vi "low energy end.vi"() -> ()   [LabVIEW 2016, in "beamline sections.lvlib"]
uses:
  beamline sections.lvlib
panel:
  out "error out":errorcluster
  out "Steerer Y":dbl format="%#_4g"
  in  "Tab Control":enum32{"Controls", "readbacks"}(tab)
  in  "Low Energy Einzel":dbl(slide) scale=30.0..50.0
  in  "Injector Image Einzel":dbl(slide) scale=30.0..50.0
  out "Low Energy Einzel Display":bool=TRUE
  out "Tank Entrance  Steerer Display":bool
  out "Low energy waist Steerer Display":bool=TRUE
  out "Injector Image Steerer display":bool
  out "Injector image Einzel Display":bool=TRUE
  in  "Tank Entrance Y2 steerer":dbl(slide) scale=-3.0..3.0
  in  "Tank Entrance Y1 steerer":dbl(slide) scale=-3.0..3.0
  in  "Tank Entrance  X steerer":dbl(slide) scale=-3.0..3.0
  in  "Low Energy Waist Y steerer":dbl(slide) scale=-1.0..1.0
  in  "Low Energy Waist  X steerer":dbl(slide) scale=-1.0..1.0
  in  "Injector Image Y steerer":dbl(slide) scale=-1.0..1.0
  in  "Injector Image X steerer":dbl(slide) scale=-1.0..1.0
  out "Low Energy Einzel Voltage":dbl format="%#.2g"
  out "Low Energy Einzel Current":dbl format="%#.2g"
  out "Tank Exit  X V":dbl format="%#.2g"
  out "Tank Exit Y #1 V":dbl format="%#.2g"
  out "Tank Exit Y #2 V":dbl format="%#.2g"
  out "Low energy waist  X V":dbl format="%#.2g"
  out "Low energy waist  Y V":dbl format="%#.2g"
  out "Inj image Einzel Current":dbl format="%#.2g"
  out "Inj image Einzel":dbl format="%#.2g"
  out "Inj Image X Voltage":dbl format="%#.2g"
  out "Inj Image Y Voltage":dbl format="%#.2g"
  in  "stop":bool
  out "LE Waist  Ion gauge Cluster":T1
  out "Tank entrance Ion gauge Cluster 1":T1
  out "Low energy   Y-":dbl format="%#_4g"
  out "Low energy   Y+":dbl format="%#_4g"
  out "Low energy   X-":dbl format="%#_4g"
  out "Low energy   X+":dbl format="%#_4g"
  out "Low energy   Y-  2":dbl format="%#_4g"
  out "Low energy   Y+  2":dbl format="%#_4g"
  out "Low energy   X-  V":dbl format="%#_4g"
  out "Low energy   X+  V":dbl format="%#_4g"
  out "Low energy waist  X+":dbl format="%#_4g"
  out "Low energy waist  Y- V":dbl format="%#_4g"
  out "Low energy waist  Y+ V":dbl format="%#_4g"
  out "Low energy waist  X- V":dbl format="%#_4g"
  out "Low energy waist  X+ V":dbl format="%#_4g"
  in  "Injector image Y  -":dbl format="%#_4g"
  in  "Injector image Y +":dbl format="%#_4g"
  in  "Injector image X  -":dbl format="%#_4g"
  in  "Injector image X +":dbl format="%#_4g"
  out "Injector image Y  -  V":dbl format="%#_4g"
  out "Injector image Y +   V":dbl format="%#_4g"
  out "Injector image X  - V":dbl format="%#_4g"
  out "Injector image X +  V":dbl format="%#_4g"
  out "Low energy   Y+ 2  V":dbl format="%#_4g"
  out "Low energy   Y- 2  V":dbl format="%#_4g"
  out "Tank entrance Cryo pump":T2
  out "Low energy   Y+  V":dbl format="%#_4g"
  out "Low energy   Y-  V":dbl format="%#_4g"
  out "Low energy waist  X-":dbl format="%#_4g"
  out "Low energy waist  Y+":dbl format="%#_4g"
  out "Low energy waist  Y-":dbl format="%#_4g"
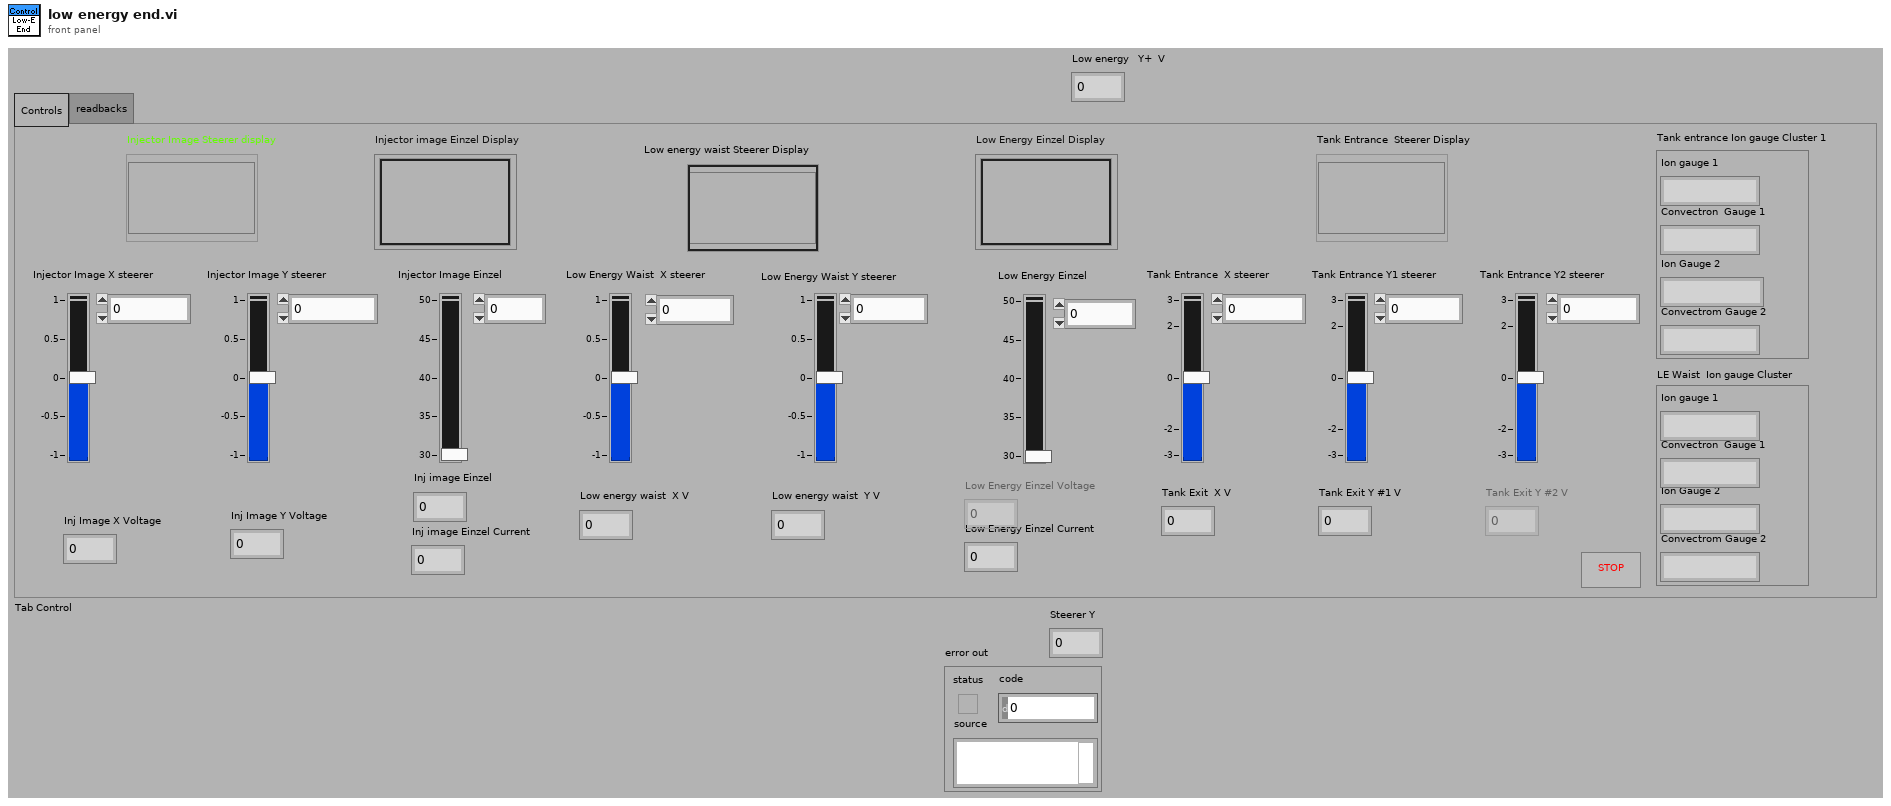
[diagram p1: front panel]
types:
  T1 = cluster{"Ion gauge 1":string, "Convectron  Gauge 1 ":string, "Ion Gauge 2":string, "Convectrom Gauge 2":string}
  T2 = cluster{"First Stage":dbl, "Second stage":dbl, "Hours since last regen":dbl, "Pump ON":bool, "Time on":dbl}
  T3 = typedef "saveload.ctl" = cluster{"OK Button":bool, "OK Button 2":bool, "OK Button 3":bool, "OK Button 4":bool}
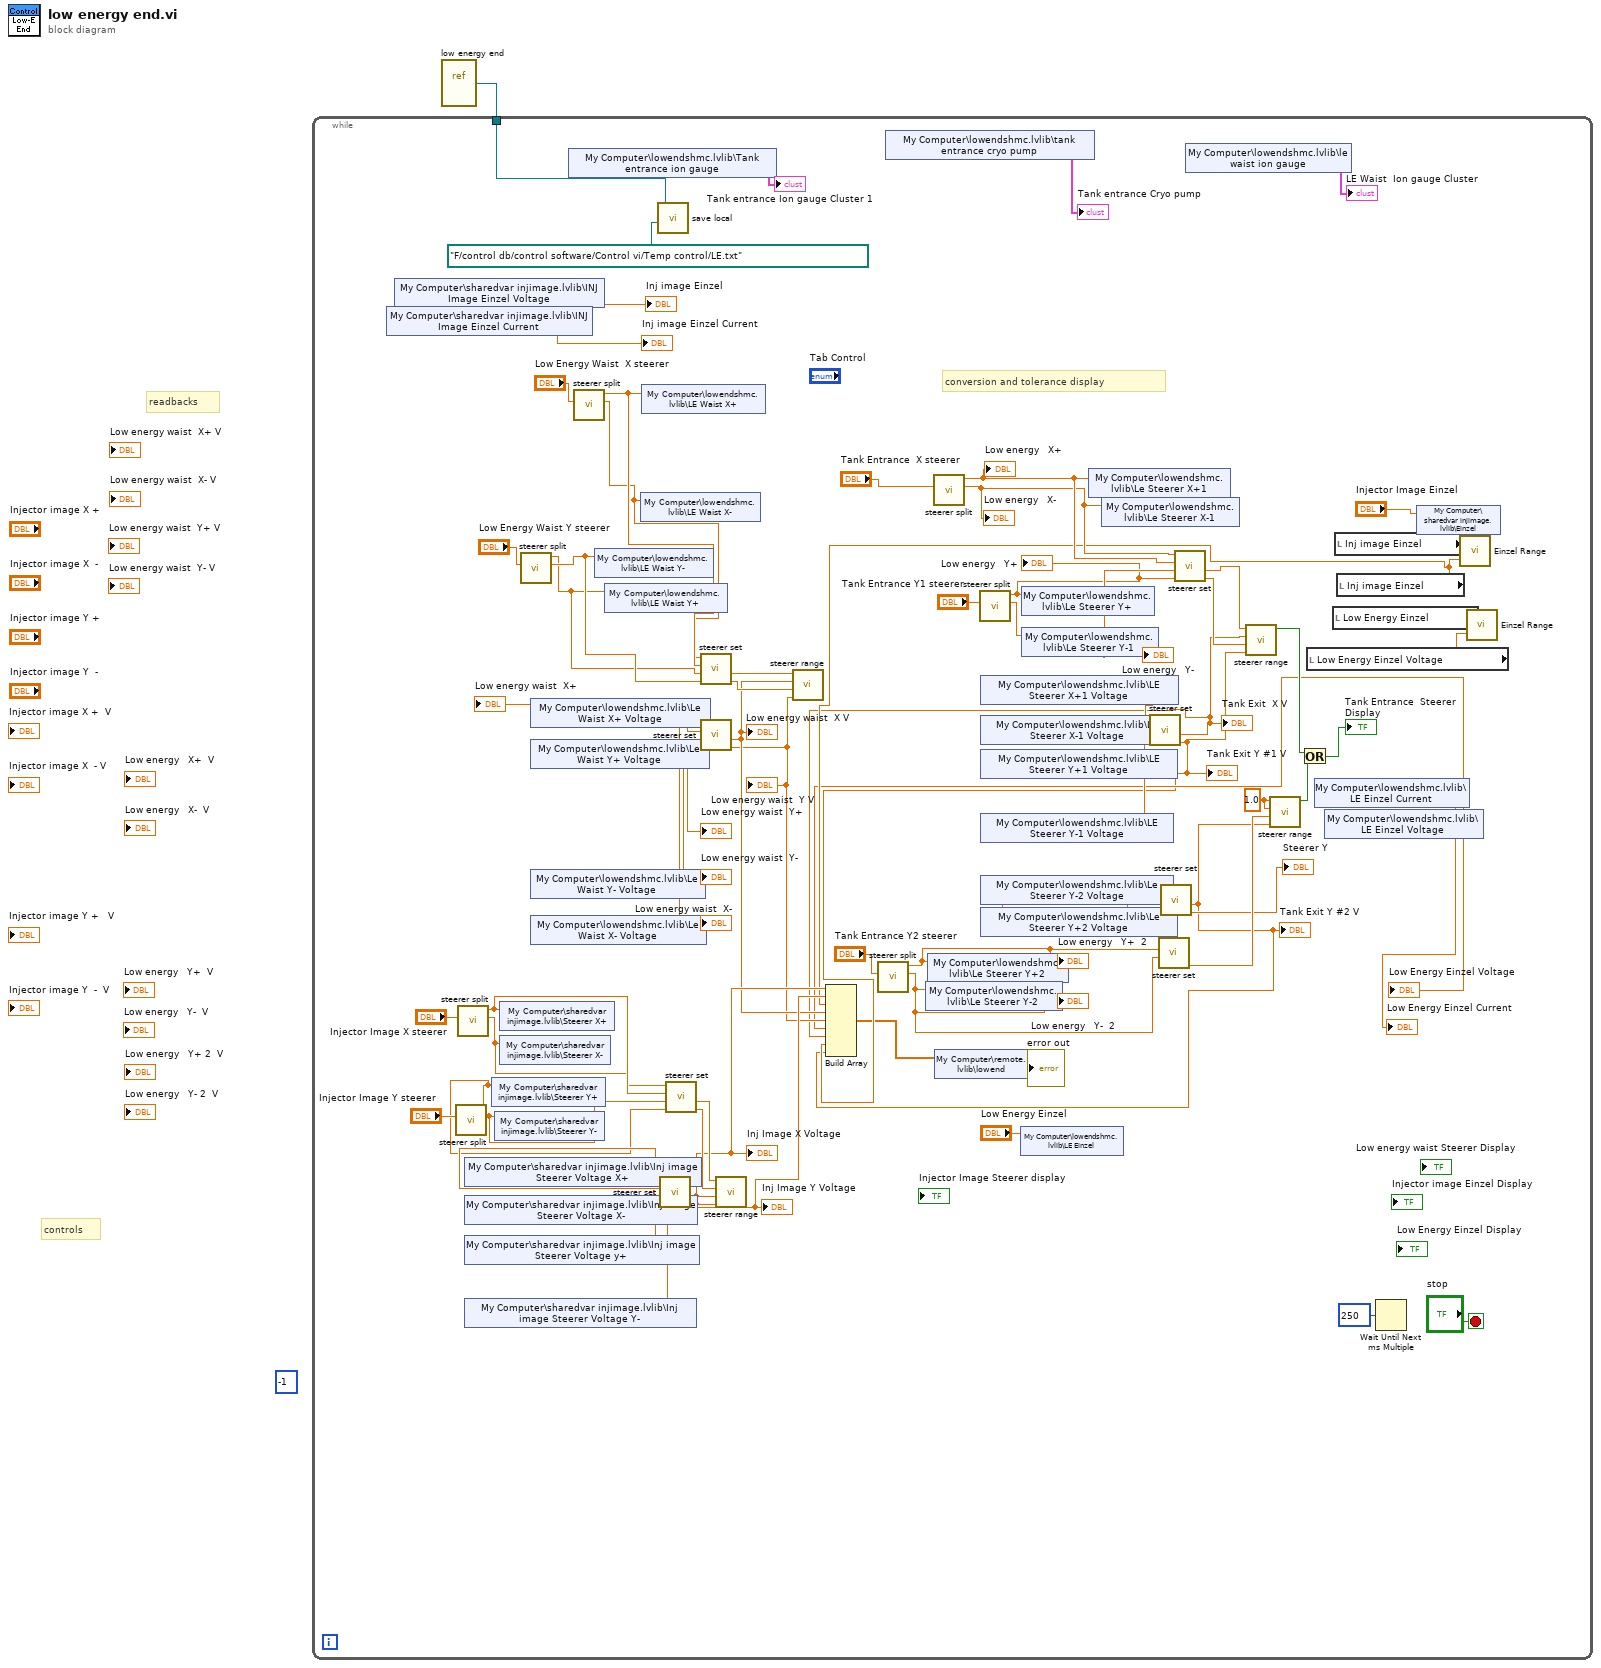
[diagram p0: block diagram]
diagram:
  (unwired) -1 ("index of element")
  # "readbacks"
  # "controls"
  n1 = vi-ref "low energy end.vi"() -> (w1:refnum<vi>)
  n2 = while {
    tunnel: w1 -> [w58]
    stop <- "stop" stop-if-true
    w66 = 1.0 ("Steerer X Set")
    # "conversion and tolerance display"
    n3 = shared-variable "My Computer\\sharedvar injimage.lvlib\\INJ Image Einzel Current"() -> (→"Inj image Einzel Current":dbl)  [unwired: 1 in, 1 out]
    n4 = shared-variable "My Computer\\sharedvar injimage.lvlib\\INJ Image Einzel Voltage"() -> (→"Inj image Einzel":dbl)  [unwired: 1 in, 1 out]
    n5 = call "steerer split.vi"("Steerer in"="Injector Image Y steerer") -> ("Steerer +"=w24:dbl, "Steerer -"=w23:dbl)  [unwired: 7 out]
    n6 = call "steerer split.vi"("Steerer in"="Injector Image X steerer") -> ("Steerer +"=w26:dbl, "Steerer -"=w25:dbl)  [unwired: 7 out]
    n7 = shared-variable "My Computer\\sharedvar injimage.lvlib\\Inj image Steerer Voltage X+"() -> (w35:dbl)  [unwired: 1 in, 1 out]
    n8 = shared-variable "My Computer\\sharedvar injimage.lvlib\\Inj image Steerer Voltage X-"() -> (w34:dbl)  [unwired: 1 in, 1 out]
    n9 = shared-variable "My Computer\\sharedvar injimage.lvlib\\Inj image Steerer Voltage y+"() -> (w33:dbl)  [unwired: 1 in, 1 out]
    n10 = shared-variable "My Computer\\sharedvar injimage.lvlib\\Inj image Steerer Voltage Y-"() -> (w36:dbl)  [unwired: 1 in, 1 out]
    n11 = shared-variable "My Computer\\sharedvar injimage.lvlib\\Steerer Y+"(w24) -> ()  [unwired: 1 in, 1 out]
    n12 = shared-variable "My Computer\\sharedvar injimage.lvlib\\Steerer Y-"(w23) -> ()  [unwired: 1 in, 1 out]
    n13 = shared-variable "My Computer\\sharedvar injimage.lvlib\\Steerer X+"(w26) -> ()  [unwired: 1 in, 1 out]
    n14 = shared-variable "My Computer\\sharedvar injimage.lvlib\\Steerer X-"(w25) -> ()  [unwired: 1 in, 1 out]
    n15 = call "steerer split.vi"("Steerer in"="Low Energy Waist Y steerer") -> ("Steerer +"=w31:dbl, "Steerer -"=w32:dbl)  [unwired: 7 out]
    n16 = shared-variable "My Computer\\lowendshmc.lvlib\\Le Waist X+ Voltage"() -> (w40:dbl)  [unwired: 1 in, 1 out]
    "Low energy waist  X+" <- w40
    n17 = shared-variable "My Computer\\lowendshmc.lvlib\\Le Waist Y+ Voltage"() -> (w38:dbl)  [unwired: 1 in, 1 out]
    "Low energy waist  Y+" <- w38
    n18 = shared-variable "My Computer\\lowendshmc.lvlib\\Le Waist Y- Voltage"() -> (w37:dbl)  [unwired: 1 in, 1 out]
    "Low energy waist  Y-" <- w37
    n19 = shared-variable "My Computer\\lowendshmc.lvlib\\Le Waist X- Voltage"() -> (w39:dbl)  [unwired: 1 in, 1 out]
    "Low energy waist  X-" <- w39
    n20 = shared-variable "My Computer\\lowendshmc.lvlib\\Tank entrance ion gauge"() -> (→"Tank entrance Ion gauge Cluster 1":cluster{string, string, string, string})  [unwired: 1 in, 1 out]
    n21 = call "steerer split.vi"("Steerer in"="Low Energy Waist  X steerer") -> ("Steerer +"=w30:dbl, "Steerer -"=w29:dbl)  [unwired: 7 out]
    n22 = shared-variable "My Computer\\lowendshmc.lvlib\\LE Waist Y-"(w32) -> ()  [unwired: 1 in, 1 out]
    n23 = shared-variable "My Computer\\lowendshmc.lvlib\\LE Waist Y+"(w31) -> ()  [unwired: 1 in, 1 out]
    n24 = shared-variable "My Computer\\lowendshmc.lvlib\\LE Waist X-"(w29) -> ()  [unwired: 1 in, 1 out]
    n25 = shared-variable "My Computer\\lowendshmc.lvlib\\LE Waist X+"(w30) -> ()  [unwired: 1 in, 1 out]
    n26 = call "save local.vi"("file path (use dialog)"=path "F:/control db/control software/Control vi/Temp control/LE.txt", "VI Refnum"=w58) -> ("Ring"=w61:T3)  [unwired: 2 out]
    n27 = call "steerer set.vi"("Injector image X  -"=w34, "Injector image X +"=w35, "Injector image Y  -"=w36, "Injector image Y +"=w33) -> ("Steerer X"=w13:dbl, "Steerer Y"=w12:dbl)  [unwired: 4 out]
    "Inj Image X Voltage" <- w13
    "Inj Image Y Voltage" <- w12
    n28 = call "steerer set.vi"("Injector image X  -"=w25, "Injector image X +"=w26, "Injector image Y  -"=w23, "Injector image Y +"=w24) -> ("Steerer X"=w72:dbl, "Steerer Y"=w73:dbl)  [unwired: 4 out]
    n29 = call "steerer set.vi"("Injector image X  -"=w29, "Injector image X +"=w30, "Injector image Y  -"=w31, "Injector image Y +"=w32) -> ("Steerer X"=w71:dbl, "Steerer Y"=w70:dbl)  [unwired: 4 out]
    n30 = call "steerer set.vi"("Injector image X  -"=w39, "Injector image X +"=w40, "Injector image Y  -"=w37, "Injector image Y +"=w38) -> ("Steerer X"=w10:dbl, "Steerer Y"=w9:dbl)  [unwired: 4 out]
    "Low energy waist  X V" <- w10
    "Low energy waist  Y V" <- w9
    n31 = call "steerer range.vi"("Steerer Y Voltage"=w12, "Steerer X Voltage"=w13, "Steerer Set Y"=w73, "Steerer X Set"=w72) -> ()  [unwired: 4 out]
    n32 = call "steerer range.vi"("Steerer Y Voltage"=w9, "Steerer X Voltage"=w70, "Steerer Set Y"=w10, "Steerer X Set"=w71) -> ()  [unwired: 4 out]
    n33 = call "steerer split.vi"("Steerer in"="Tank Entrance Y2 steerer") -> ("Steerer +"=w27:dbl, "Steerer -"=w28:dbl)  [unwired: 7 out]
    "Low energy   Y+  2" <- w27
    "Low energy   Y-  2" <- w28
    n34 = shared-variable "My Computer\\lowendshmc.lvlib\\tank entrance cryo pump"() -> (→"Tank entrance Cryo pump":T2)  [unwired: 1 in, 1 out]
    n35 = shared-variable "My Computer\\lowendshmc.lvlib\\Le Steerer Y-2"(w28) -> ()  [unwired: 1 in, 1 out]
    n36 = shared-variable "My Computer\\lowendshmc.lvlib\\Le Steerer Y+2"(w27) -> ()  [unwired: 1 in, 1 out]
    n37 = call "steerer split.vi"("Steerer in"="Tank Entrance  X steerer") -> ("Steerer +"=w20:dbl, "Steerer -"=w19:dbl)  [unwired: 7 out]
    "Low energy   X+" <- w20
    "Low energy   X-" <- w19
    n38 = call "steerer split.vi"("Steerer in"="Tank Entrance Y1 steerer") -> ("Steerer +"=w21:dbl, "Steerer -"=w22:dbl)  [unwired: 7 out]
    "Low energy   Y+" <- w21
    "Low energy   Y-" <- w22
    n39 = shared-variable "My Computer\\lowendshmc.lvlib\\LE Steerer X+1 Voltage"() -> (w47:dbl)  [unwired: 1 in, 1 out]
    n40 = shared-variable "My Computer\\lowendshmc.lvlib\\LE Steerer X-1 Voltage"() -> (w46:dbl)  [unwired: 1 in, 1 out]
    n41 = shared-variable "My Computer\\lowendshmc.lvlib\\LE Steerer Y+1 Voltage"() -> (w44:dbl)  [unwired: 1 in, 1 out]
    n42 = shared-variable "My Computer\\lowendshmc.lvlib\\LE Steerer Y-1 Voltage"() -> (w45:dbl)  [unwired: 1 in, 1 out]
    n43 = shared-variable "My Computer\\lowendshmc.lvlib\\Le Steerer Y-2 Voltage"() -> (w43:dbl)  [unwired: 1 in, 1 out]
    n44 = shared-variable "My Computer\\lowendshmc.lvlib\\Le Steerer Y+2 Voltage"() -> (w42:dbl)  [unwired: 1 in, 1 out]
    n45 = shared-variable "My Computer\\lowendshmc.lvlib\\LE Einzel"("Low Energy Einzel") -> ()  [unwired: 1 in, 1 out]
    n46 = shared-variable "My Computer\\lowendshmc.lvlib\\Le Steerer Y+"(w21) -> ()  [unwired: 1 in, 1 out]
    n47 = shared-variable "My Computer\\lowendshmc.lvlib\\Le Steerer Y-1"(w22) -> ()  [unwired: 1 in, 1 out]
    n48 = shared-variable "My Computer\\lowendshmc.lvlib\\Le Steerer X+1"(w20) -> ()  [unwired: 1 in, 1 out]
    n49 = shared-variable "My Computer\\lowendshmc.lvlib\\Le Steerer X-1"(w19) -> ()  [unwired: 1 in, 1 out]
    n50 = call "steerer set.vi"("Injector image X  -"=w46, "Injector image X +"=w47, "Injector image Y  -"=w45, "Injector image Y +"=w44) -> ("Steerer X"=w6:dbl, "Steerer Y"=w5:dbl)  [unwired: 4 out]
    "Tank Exit  X V" <- w6
    "Tank Exit Y #1 V" <- w5
    n51 = call "steerer set.vi"("Injector image Y  -"=w28, "Injector image Y +"=w27) -> ("Steerer Y"=w67:dbl)  [unwired: 2 in, 5 out]
    n52 = call "steerer set.vi"("Injector image X  -"=w43, "Injector image X +"=w42, "Injector image Y  -"=w42, "Injector image Y +"=w43) -> ("Steerer X"=w4:dbl, "Steerer Y"=→"Steerer Y":dbl)  [unwired: 4 out]
    "Tank Exit Y #2 V" <- w4
    n53 = call "steerer set.vi"("Injector image X  -"=w19, "Injector image X +"=w20, "Injector image Y  -"=w22, "Injector image Y +"=w21) -> ("Steerer X"=w69:dbl, "Steerer Y"=w68:dbl)  [unwired: 4 out]
    n54 = shared-variable "My Computer\\lowendshmc.lvlib\\le waist ion gauge"() -> (→"LE Waist  Ion gauge Cluster":cluster{string, string, string, string})  [unwired: 1 in, 1 out]
    n55 = call "steerer range.vi"("Steerer Y Voltage"=w5, "Steerer X Voltage"=w68, "Steerer Set Y"=w6, "Steerer X Set"=w69) -> ("Steerer within range"=w64:bool)  [unwired: 3 out]
    n56 = call "steerer range.vi"("Steerer Y Voltage"=w4, "Steerer X Voltage"=w67, "Steerer Set Y"=w66, "Steerer X Set"=w66) -> ("Steerer within range"=w65:bool)  [unwired: 3 out]
    n57 = Or(x=w64, y=w65) -> (x .or. y?=→"Tank Entrance  Steerer Display":bool)
    n58 = local read "Low Energy Einzel Voltage"() -> (w8:dbl)
    n59 = shared-variable "My Computer\\lowendshmc.lvlib\\LE Einzel Current"() -> (→"Low Energy Einzel Current":dbl)  [unwired: 1 in, 1 out]
    n60 = shared-variable "My Computer\\lowendshmc.lvlib\\LE Einzel Voltage"() -> (w7:dbl)  [unwired: 1 in, 1 out]
    "Low Energy Einzel Voltage" <- w7
    n61 = local read "Low Energy Einzel"() -> (w51:dbl)
    n62 = local read "Inj image Einzel"() -> (w62:dbl)
    n63 = local read "Inj image Einzel"() -> (w11:dbl)
    n64 = Build Array(w13, w12, w11, w10, w9, w7, w6, w5, w4) -> (w3:dbl[])
    n65 = shared-variable "My Computer\\remote.lvlib\\lowend"(w3) -> (error out=→"error out":errorcluster)  [unwired: 1 in]
    n66 = Wait Until Next ms Multiple(millisecond multiple=u32 250) -> ()  [unwired: 1 out]
    n67 = shared-variable "My Computer\\sharedvar injimage.lvlib\\Einzel"("Injector Image Einzel") -> ()  [unwired: 1 in, 1 out]
    n68 = call "Einzel Range.vi"("Inj image Readback"=w11, "Inj image Einzel Set"=w62) -> ()  [unwired: 2 out]
    n69 = call "Einzel Range.vi"("Inj image Readback"=w8, "Inj image Einzel Set"=w51) -> ()  [unwired: 2 out]
  }
